vi "Search position spec.vi"(10 "Image position":T1=enum."Top right", 11 "Stitch layout spec":T2) -> (3 "index of element":i32)   [LabVIEW 2020]
uses:
  Cam video sync/Typedefs/Stitch layout spec cluster.ctl
  Typedefs/Image stitching positions.ctl
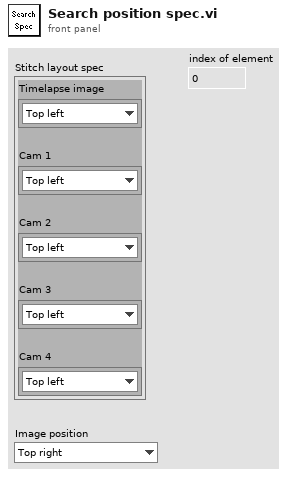
[diagram p1: front panel]
types:
  T1 = typedef "Image stitching positions.ctl" = enum16{"Top left", "Top right", "Bottom left", "Bottom right", "Not used"}
  T2 = typedef "Stitch layout spec cluster.ctl" = cluster{"Timelapse image":cluster{"Image position":T1}, "Cam 1":cluster{"Image position":T1}, "Cam 2":cluster{"Image position":T1}, "Cam 3":cluster{"Image position":T1}, "Cam 4":cluster{"Image position":T1}}
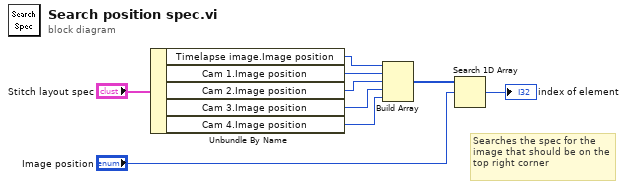
[diagram p0: block diagram]
diagram:
  # "Searches the spec for the image that should be on the top right corner"
  n1 = Unbundle By Name("Stitch layout spec") -> ("Timelapse image.Image position"=w9:T1, "Cam 1.Image position"=w6:T1, "Cam 2.Image position"=w5:T1, "Cam 3.Image position"=w4:T1, "Cam 4.Image position"=w8:T1)
  n2 = Build Array(w9, w6, w5, w4, w8) -> (w3:T1[])
  n3 = Search 1D Array(1D array=w3, element="Image position") -> (index of element=→"index of element":i32)  [unwired: 1 in]
